vi "ExecuteRobotCommandsUDP.vi"(2 "Robot Status":T1={"Left Speed (1150 to 1750)"=1500, "Right Speed (1150 to 1750)"=1500, "Robot Heading"=0, "UDP Transmitting Port"=0, "UDP Receiving Port"=0, "Robot Symbol"=""}, 3 "Robot Position":i32[](array[numeric])) -> (0 "Updated Robot Heading":i32, 1 "Updated Robot Position":i32[](array[numeric]))   [LabVIEW 2012]
panel:
  in  "Use Old":bool=TRUE
  out "Scaled Right":i32
  out "Scaled Left":i32
  out "Robot Y":i32
  out "Robot X":i32
  in  "upper limit":i32=10
  # "1150 to 1750 is no longer reflected in code.\nInstead, 1000 to 2000."
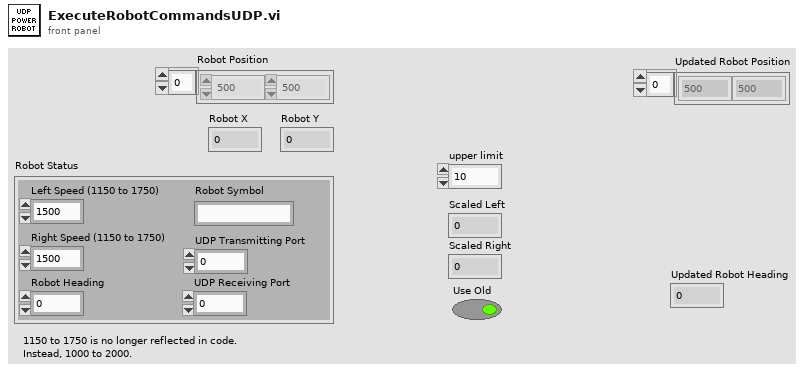
[diagram p1: front panel]
types:
  T1 = cluster{"Left Speed (1150 to 1750)":i32, "Right Speed (1150 to 1750)":i32, "Robot Heading":i32, "UDP Transmitting Port":i32, "UDP Receiving Port":i32, "Robot Symbol":string}
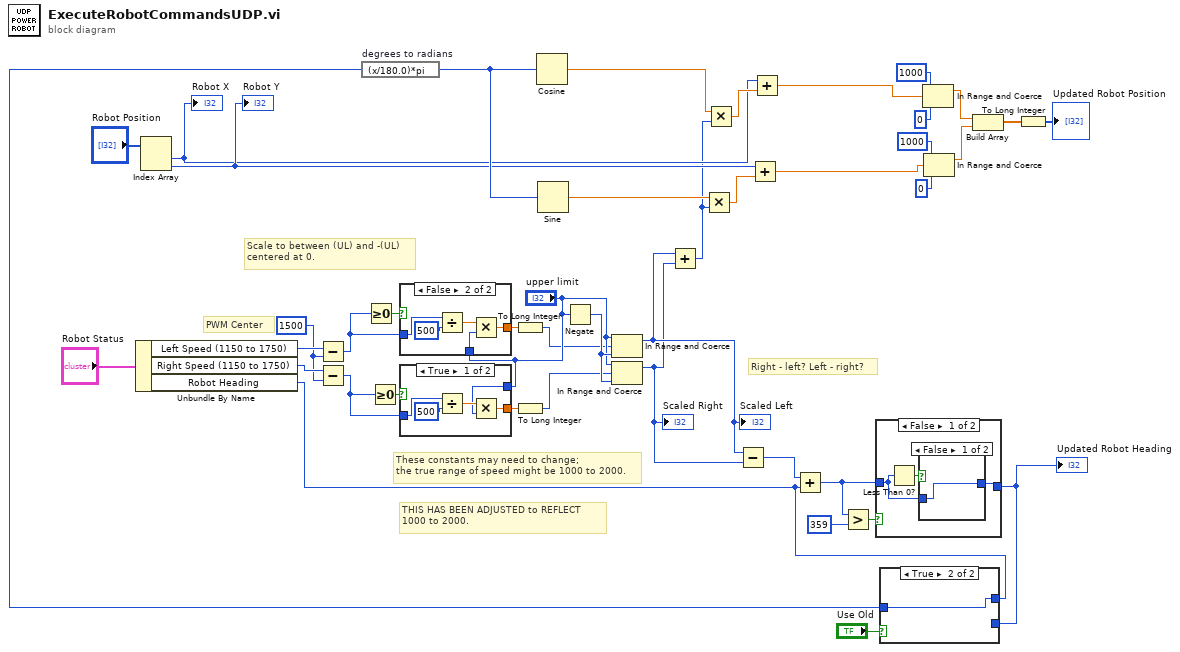
[diagram p0: block diagram]
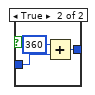
[diagram p3: hidden frame]
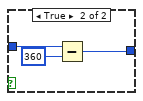
[diagram p4: hidden frame]
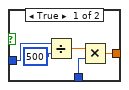
[diagram p5: hidden frame]
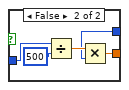
[diagram p6: hidden frame]
diagram:
  w31 = 1500 ("y")
  # "THIS HAS BEEN ADJUSTED to REFLECT\n1000 to 2000."
  # "These constants may need to change;\nthe true range of speed might be 1000 to 2000."
  # "Right - left? Left - right?"
  # "PWM Center"
  # "Scale to between (UL) and -(UL)\ncentered at 0."
  n1 = Unbundle By Name("Robot Status") -> ("Left Speed (1150 to 1750)"=w33:i32, "Right Speed (1150 to 1750)"=w32:i32, "Robot Heading"=w2:i32)
  n2 = Index Array(array="Robot Position") -> (element #1=w12:i32, element #2=w14:i32)  [unwired: 2 in]
  "Robot X" <- w12
  "Robot Y" <- w14
  n3 = Subtract(x=w33, y=w31) -> (x-y=w25:i32)
  n4 = Subtract(x=w32, y=w31) -> (x-y=w29:i32)
  n5 = Greater Or Equal To 0?(x=w25) -> (x >= 0?=w26:bool)
  n6 = Greater Or Equal To 0?(x=w29) -> (x >= 0?=w30:bool)
  n7 = case shown="False" w26 {
    tunnel: w25 -> [w48 w53]
    tunnel: "upper limit" -> [w45 w50]
    tunnel: [w44 w49] -> w27
    frame True {
      n8 = Divide(x=w48, y=500) -> (x/y=w46:dbl)
      n9 = Multiply(x=w46, y=w45) -> (x*y=w44:dbl)
    }
    frame False {
      n10 = Divide(x=w53, y=500) -> (x/y=w51:dbl)
      n11 = Multiply(x=w51, y=w50) -> (x*y=w49:dbl)
    }
  }
  n12 = case shown="True" w30 {
    tunnel: w29 -> [w58 w63]
    tunnel: "upper limit" -> [w55 w60]
    tunnel: [w54 w59] -> w28
    frame True {
      n13 = Divide(x=w58, y=500) -> (x/y=w56:dbl)
      n14 = Multiply(x=w56, y=w55) -> (x*y=w54:dbl)
    }
    frame False {
      n15 = Divide(x=w63, y=500) -> (x/y=w61:dbl)
      n16 = Multiply(x=w61, y=w60) -> (x*y=w59:dbl)
    }
  }
  n17 = To Long Integer(number=w27) -> (32bit integer=w23:i32)
  n18 = To Long Integer(number=w28) -> (32bit integer=w22:i32)
  n19 = Negate(x="upper limit") -> (-x=w35:i32)
  n20 = In Range and Coerce(upper limit="upper limit", x=w23, lower limit=w35) -> (coerced(x)=w7:i32)  [unwired: 1 out]
  "Scaled Left" <- w7
  n21 = In Range and Coerce(upper limit="upper limit", x=w22, lower limit=w35) -> (coerced(x)=w6:i32)  [unwired: 1 out]
  "Scaled Right" <- w6
  n22 = Add(x=w7, y=w6) -> (x+y=w10:i32)
  n23 = Subtract(x=w7, y=w6) -> (x-y=w21:i32)
  n24 = Add(x=w21, y=w2) -> (x+y=w18:i32)
  n25 = Greater?(x=w18, y=359) -> (0:w20:bool)
  n26 = case shown="False" w20 {
    tunnel: w18 -> [w64 w73]
    tunnel: [w65 w71] -> w3
    frame False {
      n27 = Less Than 0?(x=w64) -> (x < 0?=w66:bool)
      n28 = case shown="False" w66 {
        tunnel: [w67 w70] -> w65
        tunnel: w64 -> [w67 w69]
        frame False {
        }
        frame True {
          n29 = Add(x=360, y=w69) -> (x+y=w70:i32)
        }
      }
    }
    frame True {
      n30 = Subtract(x=w73, y=360) -> (x-y=w71:i32)
    }
  }
  "Updated Robot Heading" <- w3
  n31 = case shown="True" "Use Old" {
    tunnel: [w74 w75] -> w4
    tunnel: w2 -> [_ w75]
    tunnel: w3 -> [w74 _]
    frame False {
    }
    frame True {
    }
  }
  n32 = expression code="(x/180.0)*pi" "degrees to radians"(w4) -> (w17:i32)
  n33 = Cosine(x=w17) -> (cos(x)=w11:dbl)
  n34 = Sine(x=w17) -> (sin(x)=w16:dbl)
  n35 = Multiply(x=w16, y=w10) -> (x*y=w15:dbl)
  n36 = Multiply(x=w11, y=w10) -> (x*y=w13:dbl)
  n37 = Add(x=w14, y=w15) -> (x+y=w8:dbl)
  n38 = Add(x=w12, y=w13) -> (x+y=w9:dbl)
  n39 = In Range and Coerce(upper limit=1000, x=w9, lower limit=0) -> (coerced(x)=w36:dbl)  [unwired: 1 out]
  n40 = In Range and Coerce(upper limit=1000, x=w8, lower limit=0) -> (coerced(x)=w37:dbl)  [unwired: 1 out]
  n41 = Build Array(w36, w37) -> (w42:dbl[])
  n42 = To Long Integer(number=w42) -> (32bit integer=→"Updated Robot Position":i32[])
